vi "Regenerate ID.vi"(8 "error in (no error)":errorcluster, 11 "Session in":refnum<class "Session.lvclass">) -> (0 "error out":errorcluster, 1 "Hashed ID":string, 2 "ID":string, 3 "Session out":refnum<class "Session.lvclass">)   [LabVIEW 2020, in "HTTP Server.lvlib" / "Session.lvclass"]
uses:
  Session.lvclass
  lv-web-crypto/lv-crypto/Crypto/Crypto.lvlib
  lv-web-crypto/lv-json/JSON/JSON.lvlib
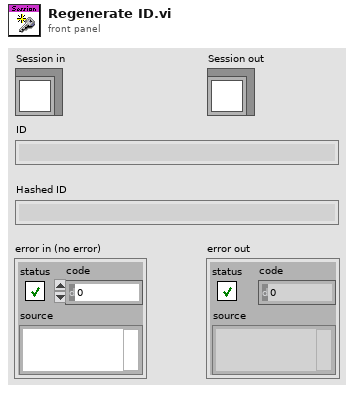
[diagram p1: front panel]
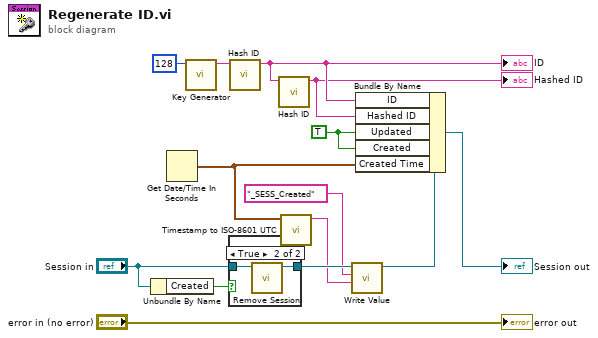
[diagram p0: block diagram]
diagram:
  w6 = TRUE ("Updated")
  n1 = Unbundle By Name("Session in") -> ("Created"=w7:bool)
  n2 = Get Date/Time In Seconds() -> (seconds since 1Jan1904=w2:timestamp)
  n3 = call "Key Generator.vi"("Bits (256)"=128) -> ("Key"=w8:string)  [unwired: 9 in, 1 out]
  n4 = case shown="True" w7 {
    tunnel: "Session in" -> [w15 w17]
    tunnel: [w15 w16] -> w5
    frame False {
    }
    frame True {
      n5 = call-dynamic "Remove Session.vi"("Session in"=w17) -> ("Session out"=w16:refnum<class "Session.lvclass">)  [unwired: 9 in, 1 out]
    }
  }
  n6 = call "Hash ID.vi"("ID"=w8) -> ("Hashed ID"=w12:string)  [unwired: 10 in]
  "ID" <- w12
  n7 = call "Hash ID.vi"("ID"=w12) -> ("Hashed ID"=w11:string)  [unwired: 10 in]
  "Hashed ID" <- w11
  n8 = call "Timestamp to ISO-8601 UTC.vi"("Time Stamp"=w2) -> ("ISO 8601 UTC"=w1:string)  [unwired: 10 in]
  n9 = call "Write Value.vi"("Value"=w1, "Name"="_SESS_Created", "Session in"=w5) -> ("Session out"=w4:refnum<class "Session.lvclass">)  [unwired: 6 in, 2 out]
  n10 = Bundle By Name(cluster=w4, "ID"=w12, "Hashed ID"=w11, "Updated"=w6, "Created"=w6, "Created Time"=w2) -> (→"Session out":refnum<class "Session.lvclass">)
  "error out" <- "error in (no error)"
